vi "serial.Init.vi"(8 "error in":errorcluster, 11 "VISA Refnum in":refnum<visa-resource-name>="COM5") -> (0 "error out":errorcluster, 1 "connected":bool, 2 "VISA out":refnum<visa-resource-name>)   [LabVIEW 2020]
uses:
  6e6c0c51-725f-4bbb-aef5-0ff21f71116e.vi
  fbe725bf-f9b1-496f-8713-48bec69dc5a8.vi
  <vilib>/Instr/_visa.llb/VISA Configure Serial Port (Instr).vi
panel:
  out "msg":string
  out "read buffer":string
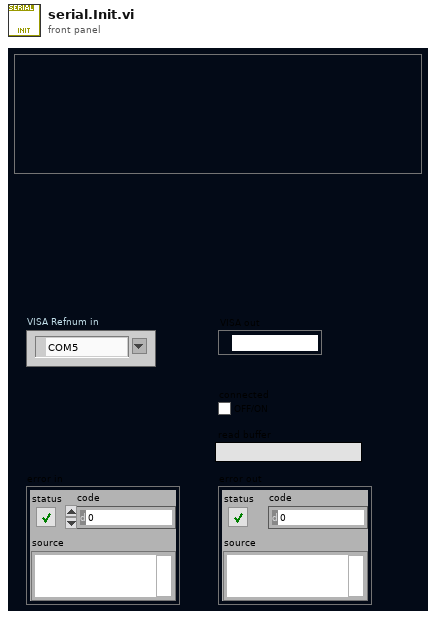
[diagram p1: front panel]
types:
  T1 = cluster{"baud rate":u32, "data bits":u16, "parity":enum16{"None", "Odd", "Even", "Mark", "Space"}, "stop bits":u16, "flow control":u16}
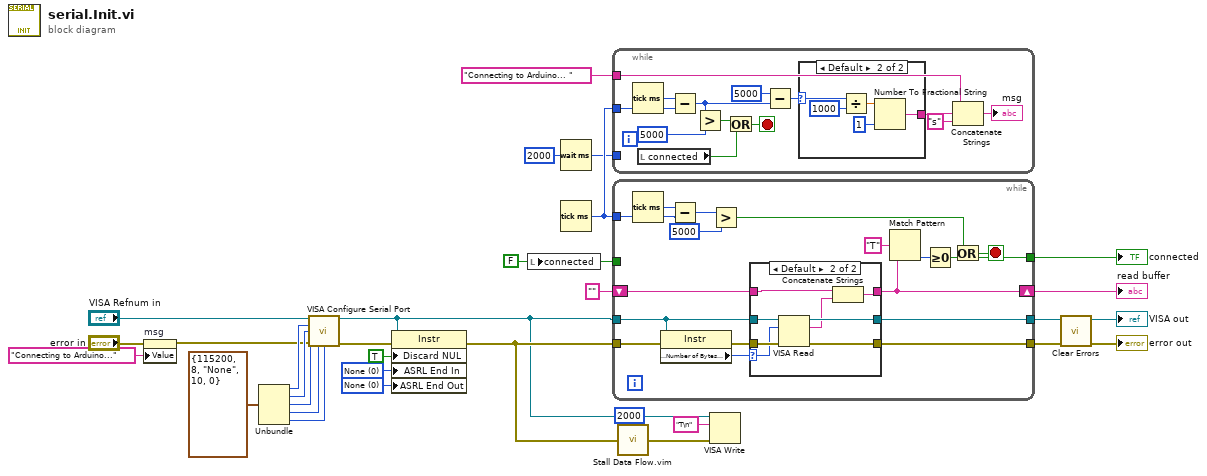
[diagram p0: block diagram]
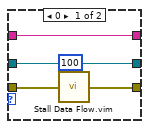
[diagram p2: hidden frame]
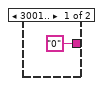
[diagram p3: hidden frame]
diagram:
  w11 = FALSE ("connected")
  w20 = u16 0 items=["None", "Last Bit", "TermChar", "Break"] ("End Mode for Writes")
  w21 = u16 0 items=["None", "Last Bit", "TermChar"] ("End Mode for Reads")
  n1 = property on="msg" class="Str"(error in="error in", "Value"="Connecting to Arduino..." ("msg")) -> (error out=w7:errorcluster)  [unwired: 1 in, 1 out]
  n2 = Unbundle(T1 {"baud rate"=115200, "data bits"=8, "parity"=enum."None", "stop bits"=10, "flow control"=0} ("Serial Settings")) -> ("baud rate"=w27:u32, "data bits"=w26:u16, "parity"=w25:enum16{"None", "Odd", "Even", "Mark", "Space"}, "stop bits"=w24:u16, "flow control"=w23:u16)
  n3 = call-poly "VISA Configure Serial Port"("VISA resource name"="VISA Refnum in", "baud rate (9600)"=w27, "data bits (8)"=w26, "parity (0:none)"=w25, "error in (no error)"=w7, "stop bits (10: 1 bit)"=w24, "flow control (0:none)"=w23) -> ("VISA resource name out"=w4:refnum<visa-resource-name>, "error out"=w19:errorcluster)  [unwired: 2 in, 5 out]
  n4 = property class="Instr"(reference=w4, error in=w19, "Discard NUL"=TRUE ("Serial Settings:Discard NUL Characters"), "ASRL End In"=w21, "ASRL End Out"=w20) -> (error out=w5:errorcluster)  [unwired: 1 out]
  n5 = local write "connected"(w11) -> ()
  n6 = Wait (ms)(milliseconds to wait=u32 2000) -> (millisecond timer value=w1:u32)
  n7 = Tick Count (ms)() -> (millisecond timer value=w3:u32)
  n8 = while {
    tunnel: w3 -> [w39]
    tunnel: "Connecting to Arduino... " -> [w34]
    tunnel: w1 -> [_]
    stop <- w33 stop-if-true
    n9 = Tick Count (ms)() -> (millisecond timer value=w40:u32)
    n10 = local read "connected"() -> (w32:bool)
    n11 = Subtract(x=w40, y=w39) -> (x-y=w37:u32)
    n12 = Greater?(x=w37, y=u32 5000) -> (0:w36:bool)
    n13 = Or(x=w36, y=w32) -> (x .or. y?=w33:bool)
    n14 = Subtract(x=u32 5000 ("y"), y=w37) -> (x-y=w31:u32)
    n15 = case shown="Default" w31 {
      selector: w31 -> [_ w45]
      tunnel: ["0" w47] -> w35
      frame 3001.. {
      }
      frame Default {
        n16 = Divide(x=w45, y=u32 1000) -> (x/y=w49:dbl)
        n17 = Number To Fractional String(number=w49, precision (6)=i16 1) -> (F-format string=w47:string)  [unwired: 2 in]
      }
    }
    n18 = Concatenate Strings(w34, w35, "s" ("string")) -> (→"msg":string)
  }
  n19 = while {
    tunnel: w5 -> [w64]
    tunnel: w4 -> [w53]
    tunnel: w3 -> [w59]
    shift-right: [w62] -> w15
    shift-left: "" ("read buffer") -> [w63]
    tunnel: [w56] -> w30
    tunnel: [w54] -> w10
    tunnel: [w52] -> w16
    tunnel: w11 -> [_]
    stop <- w57 stop-if-true
    n20 = Tick Count (ms)() -> (millisecond timer value=w60:u32)
    n21 = property class="Instr"(reference=w53, error in=w64) -> (error out=w66:errorcluster, "Serial Settings:Number of Bytes at Serial Port"=w65:u32)  [unwired: 1 out]
    n22 = Subtract(x=w60, y=w59) -> (x-y=w51:u32)
    n23 = Greater?(x=w51, y=u32 5000) -> (0:w55:bool)
    n24 = case shown="Default" w65 {
      selector: w65 -> [_ w75]
      tunnel: [w69 w79] -> w54
      tunnel: [w70 w78] -> w56
      tunnel: w66 -> [w71 w77]
      tunnel: w53 -> [w70 w76]
      tunnel: w63 -> [w67 w72]
      tunnel: [w67 w73] -> w62
      frame 0 {
        n25 = call "Stall Data Flow.vim"("value in"=w71, "milliseconds to wait"=u32 100) -> ("value out"=w69:errorcluster)  [unwired: 1 out]
      }
      frame Default {
        n26 = VISA Read(VISA resource name=w76, byte count=w75, error in (no error)=w77) -> (VISA resource name out=w78:refnum<visa-resource-name>, read buffer=w74:string, error out=w79:errorcluster)  [unwired: 1 out]
        n27 = Concatenate Strings(w72, w74) -> (w73:string)
      }
    }
    n28 = Match Pattern(string=w62, regular expression="T") -> (offset past match=w61:i32)  [unwired: 1 in, 3 out]
    n29 = Greater Or Equal To 0?(x=w61) -> (x >= 0?=w52:bool)
    n30 = Or(x=w55, y=w52) -> (x .or. y?=w57:bool)
  }
  "VISA out" <- w30
  "connected" <- w16
  "read buffer" <- w15
  n31 = call "Stall Data Flow.vim"("value in"=w5, "milliseconds to wait"=u32 2000) -> ("value out"=w18:errorcluster)  [unwired: 1 out]
  n32 = VISA Write(VISA resource name=w4, write buffer="T\n" ("String"), error in (no error)=w18) -> ()  [unwired: 3 out]
  n33 = call <vilib>:"Clear Errors.vi"("error in (no error)"=w10) -> ("error out"=→"error out":errorcluster)  [unwired: 5 in, 1 out]
